vi "Finish.vi"   [LabVIEW 2016]
doc: "This VI is called just before exiting. It is expected to close I/O refnum, save collected data, etc."
uses:
  <vilib>/Rock Robotics/WPI/Utilities/WPI_GetSetVariantRefNum.vi
  <vilib>/Rock Robotics/WPI/Ultrasonic/WPI_SonarMB1010AnalogRefNum Registry Get.vi
  <vilib>/Rock Robotics/WPI/Ultrasonic/WPI_SonarMB1010AnalogClose.vi
types:
  T1 = typedef "WPI_SonarMB1010AnalogDeviceRef.ctl" = cluster{"AIDeviceRef":T2, "Scaling factor (V/in)":dbl, "Average Bits":u8}
  T2 = typedef "WPI_AnalogChannelDevRef.ctl" = cluster{"DevStatus":errorcluster, "Analog Channel":T3}
  T3 = typedef "FPGA_AIChannel.ctl" = enum8{"AI 0", "AI 1", "AI 2", "AI 3", "AI MXP 0", "AI MXP 1", "AI MXP 2", "AI MXP 3", "Invalid"}
  T4 = typedef "WPI_JoystickDevRef.ctl" = cluster{"Device":T5}
  T5 = typedef "WPI_JoystickDeviceEnum.ctl" = enum16{"USB 0", "USB 1", "USB 2", "USB 3", "USB 4", "USB 5"}
  T6 = typedef "WPI_RobotDriveDevRef.ctl" = cluster{"DevStatus":errorcluster, "Motors[]":T7[], "Square Inputs":bool, "Max Output":dbl}
  T7 = typedef "WPI_MotorControlDeviceRef.ctl" = cluster{"DeviceStatus":errorcluster, "Type":T8, "PWM":cluster{"PWM Channel":T9, "DeadBand":T10}, "CAN":cluster{"Device Number":u8, "SetOutput VI Ref":variant, "GetOutput VI Ref":variant, "Enable VI Ref":variant, "Disable VI Ref":variant, "Data":variant}, "Invert":bool}
  T8 = typedef "WPI_MotorControlType.ctl" = enum16{"PWM", "CAN"}
  T9 = typedef "FPGA_DIOPWMChannel.ctl" = enum8{"PWM 0", "PWM 1", "PWM 2", "PWM 3", "PWM 4", "PWM 5", "PWM 6", "PWM 7", "PWM 8", "PWM 9", "PWM MXP 0", "PWM MXP 1", "PWM MXP 2", "PWM MXP 3", "PWM MXP 4", "PWM MXP 5", "PWM MXP 6", "PWM MXP 7", "PWM MXP 8", "PWM MXP 9", "Invalid"}
  T10 = typedef "WPI_PWMDeadband.ctl" = cluster{"Name":string, "maxPositivePwm":i32, "minPositivePwm":i32, "centerPwm":i32, "maxNegativePwm":i32, "minNegativePwm":i32, "angularRange":u16}
  T11 = typedef "WPI_SwitchDevRef.ctl" = cluster{"DevStatus":errorcluster, "DIO Channel":T12, "CntIndex":T13, "Normally Closed":bool}
  T12 = typedef "FPGA_DIOChannel.ctl" = enum8{"DIO 0", "DIO 1", "DIO 2", "DIO 3", "DIO 4", "DIO 5", "DIO 6", "DIO 7", "DIO 8", "DIO 9", "DIO MXP 0", "DIO MXP 1", "DIO MXP 2", "DIO MXP 3", "DIO MXP 4", "DIO MXP 5", "DIO MXP 6", "DIO MXP 7", "DIO MXP 8", "DIO MXP 9", "DIO MXP 10", "DIO MXP 11", "DIO MXP 12", "DIO MXP 13", "DIO MXP 14", "DIO MXP 15", "SPI Port CS1", "SPI Port CS2", "SPI Port CS3", "SPI Port MISO", "SPI Port MOSI", "Invalid"}
  T13 = typedef "FPGA_CounterCtrSystemIndex.ctl" = enum8{"Ctr 0", "Ctr 1", "Ctr 2", "Ctr 3", "Ctr 4", "Ctr 5", "Ctr 6", "Ctr 7", "Invalid"}
  T14 = typedef "WPI_DigitalInputDevRef.ctl" = cluster{"DevStatus":errorcluster, "DIO Channel":T12}
  T15 = typedef "WPI_ServoDeviceRef.ctl" = cluster{"DeviceStatus":errorcluster, "PWM Channel":T9, "DeadBand":T10}
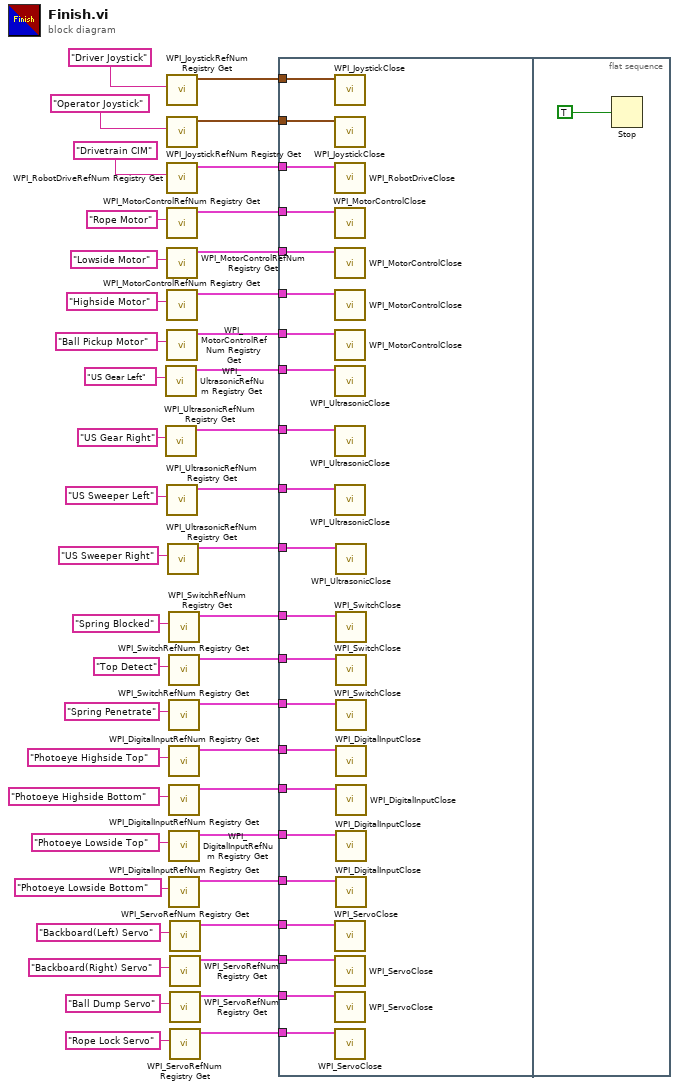
[diagram p0: block diagram]
diagram:
  n1 = call-poly <vilib>:"WPI_UltrasonicRefNum Registry Get.vi"("refnum name"="US Gear Left") -> ("SonarMB1010AnalogDevRef"=w30:T1)  [unwired: 9 in, 1 out]
  n2 = call-poly <vilib>:"WPI_UltrasonicRefNum Registry Get.vi"("refnum name"="US Gear Right") -> ("SonarMB1010AnalogDevRef"=w29:T1)  [unwired: 9 in, 1 out]
  n3 = call <vilib>:"WPI_JoystickRefNum Registry Get.vi"("refnum name"="Driver Joystick") -> ("JoystickDevRef"=w41:T4)  [unwired: 1 in, 9 out]
  n4 = call <vilib>:"WPI_JoystickRefNum Registry Get.vi"("refnum name"="Operator Joystick") -> ("JoystickDevRef"=w39:T4)  [unwired: 1 in, 9 out]
  n5 = call <vilib>:"WPI_RobotDriveRefNum Registry Get.vi"("refnum name"="Drivetrain CIM") -> ("RobotDriveDevRef"=w42:T6)  [unwired: 1 in, 9 out]
  n6 = call <vilib>:"WPI_MotorControlRefNum Registry Get.vi"("refnum name"="Rope Motor") -> ("MotorControlDevRef"=w34:T7)  [unwired: 9 in, 1 out]
  n7 = call <vilib>:"WPI_MotorControlRefNum Registry Get.vi"("refnum name"="Lowside Motor") -> ("MotorControlDevRef"=w33:T7)  [unwired: 9 in, 1 out]
  n8 = call <vilib>:"WPI_MotorControlRefNum Registry Get.vi"("refnum name"="Highside Motor") -> ("MotorControlDevRef"=w32:T7)  [unwired: 9 in, 1 out]
  n9 = call <vilib>:"WPI_MotorControlRefNum Registry Get.vi"("refnum name"="Ball Pickup Motor") -> ("MotorControlDevRef"=w31:T7)  [unwired: 9 in, 1 out]
  n10 = call-poly <vilib>:"WPI_UltrasonicRefNum Registry Get.vi"("refnum name"="US Sweeper Left") -> ("SonarMB1010AnalogDevRef"=w28:T1)  [unwired: 9 in, 1 out]
  n11 = call-poly <vilib>:"WPI_UltrasonicRefNum Registry Get.vi"("refnum name"="US Sweeper Right") -> ("SonarMB1010AnalogDevRef"=w27:T1)  [unwired: 9 in, 1 out]
  n12 = call <vilib>:"WPI_SwitchRefNum Registry Get.vi"("refnum name"="Spring Blocked") -> ("SwitchDevRef"=w22:T11)  [unwired: 9 in, 1 out]
  n13 = call <vilib>:"WPI_SwitchRefNum Registry Get.vi"("refnum name"="Top Detect") -> ("SwitchDevRef"=w21:T11)  [unwired: 9 in, 1 out]
  n14 = call <vilib>:"WPI_SwitchRefNum Registry Get.vi"("refnum name"="Spring Penetrate") -> ("SwitchDevRef"=w20:T11)  [unwired: 9 in, 1 out]
  n15 = call <vilib>:"WPI_DigitalInputRefNum Registry Get.vi"("refnum name"="Photoeye Highside Top") -> ("DigitalInputDevRef"=w16:T14)  [unwired: 9 in, 1 out]
  n16 = call <vilib>:"WPI_DigitalInputRefNum Registry Get.vi"("refnum name"="Photoeye Highside Bottom") -> ("DigitalInputDevRef"=w15:T14)  [unwired: 9 in, 1 out]
  n17 = call <vilib>:"WPI_DigitalInputRefNum Registry Get.vi"("refnum name"="Photoeye Lowside Top") -> ("DigitalInputDevRef"=w14:T14)  [unwired: 9 in, 1 out]
  n18 = call <vilib>:"WPI_DigitalInputRefNum Registry Get.vi"("refnum name"="Photoeye Lowside Bottom") -> ("DigitalInputDevRef"=w9:T14)  [unwired: 9 in, 1 out]
  n19 = call <vilib>:"WPI_ServoRefNum Registry Get.vi"("refnum name"="Backboard(Left) Servo") -> ("ServoDeviceRef"=w8:T15)  [unwired: 9 in, 1 out]
  n20 = call <vilib>:"WPI_ServoRefNum Registry Get.vi"("refnum name"="Backboard(Right) Servo") -> ("ServoDeviceRef"=w7:T15)  [unwired: 9 in, 1 out]
  n21 = call <vilib>:"WPI_ServoRefNum Registry Get.vi"("refnum name"="Ball Dump Servo") -> ("ServoDeviceRef"=w6:T15)  [unwired: 9 in, 1 out]
  n22 = call <vilib>:"WPI_ServoRefNum Registry Get.vi"("refnum name"="Rope Lock Servo") -> ("ServoDeviceRef"=w5:T15)  [unwired: 9 in, 1 out]
  n23 = flat-sequence {
    tunnel: w42 -> [w66]
    tunnel: w41 -> [w65]
    tunnel: w39 -> [w64]
    tunnel: w34 -> [w63]
    tunnel: w33 -> [w62]
    tunnel: w32 -> [w61]
    tunnel: w31 -> [w60]
    tunnel: w30 -> [w59]
    tunnel: w29 -> [w58]
    tunnel: w28 -> [w57]
    tunnel: w27 -> [w56]
    tunnel: w22 -> [w55]
    tunnel: w21 -> [w54]
    tunnel: w20 -> [w53]
    tunnel: w16 -> [w52]
    tunnel: w15 -> [w51]
    tunnel: w14 -> [w50]
    tunnel: w9 -> [w49]
    tunnel: w8 -> [w48]
    tunnel: w7 -> [w47]
    tunnel: w6 -> [w46]
    tunnel: w5 -> [w45]
    frame #0 {
      n24 = call <vilib>:"WPI_JoystickClose.vi"("JoystickDevRef"=w65) -> ()  [unwired: 11 out]
      n25 = call <vilib>:"WPI_JoystickClose.vi"("JoystickDevRef"=w64) -> ()  [unwired: 11 out]
      n26 = call <vilib>:"WPI_RobotDriveClose.vi"("RobotDriveDevRef"=w66) -> ()  [unwired: 1 in, 10 out]
      n27 = call <vilib>:"WPI_MotorControlClose.vi"("MotorControlDevRef"=w63) -> ()  [unwired: 10 in, 1 out]
      n28 = call <vilib>:"WPI_MotorControlClose.vi"("MotorControlDevRef"=w62) -> ()  [unwired: 10 in, 1 out]
      n29 = call <vilib>:"WPI_MotorControlClose.vi"("MotorControlDevRef"=w61) -> ()  [unwired: 10 in, 1 out]
      n30 = call <vilib>:"WPI_MotorControlClose.vi"("MotorControlDevRef"=w60) -> ()  [unwired: 10 in, 1 out]
      n31 = call-poly <vilib>:"WPI_UltrasonicClose.vi"("SonarMB1010AnalogDevRef"=w59) -> ()  [unwired: 10 in, 1 out]
      n32 = call-poly <vilib>:"WPI_UltrasonicClose.vi"("SonarMB1010AnalogDevRef"=w58) -> ()  [unwired: 10 in, 1 out]
      n33 = call-poly <vilib>:"WPI_UltrasonicClose.vi"("SonarMB1010AnalogDevRef"=w57) -> ()  [unwired: 10 in, 1 out]
      n34 = call <vilib>:"WPI_ServoClose.vi"("ServoDeviceRef"=w48) -> ()  [unwired: 10 in, 1 out]
      n35 = call <vilib>:"WPI_ServoClose.vi"("ServoDeviceRef"=w47) -> ()  [unwired: 10 in, 1 out]
      n36 = call <vilib>:"WPI_ServoClose.vi"("ServoDeviceRef"=w46) -> ()  [unwired: 10 in, 1 out]
      n37 = call <vilib>:"WPI_ServoClose.vi"("ServoDeviceRef"=w45) -> ()  [unwired: 10 in, 1 out]
      n38 = call-poly <vilib>:"WPI_UltrasonicClose.vi"("SonarMB1010AnalogDevRef"=w56) -> ()  [unwired: 10 in, 1 out]
      n39 = call <vilib>:"WPI_SwitchClose.vi"("SwitchDevRef"=w55) -> ()  [unwired: 10 in, 1 out]
      n40 = call <vilib>:"WPI_SwitchClose.vi"("SwitchDevRef"=w54) -> ()  [unwired: 10 in, 1 out]
      n41 = call <vilib>:"WPI_SwitchClose.vi"("SwitchDevRef"=w53) -> ()  [unwired: 10 in, 1 out]
      n42 = call <vilib>:"WPI_DigitalInputClose.vi"("DigitalInputDevRef"=w52) -> ()  [unwired: 10 in, 1 out]
      n43 = call <vilib>:"WPI_DigitalInputClose.vi"("DigitalInputDevRef"=w51) -> ()  [unwired: 10 in, 1 out]
      n44 = call <vilib>:"WPI_DigitalInputClose.vi"("DigitalInputDevRef"=w50) -> ()  [unwired: 10 in, 1 out]
      n45 = call <vilib>:"WPI_DigitalInputClose.vi"("DigitalInputDevRef"=w49) -> ()  [unwired: 10 in, 1 out]
    }
    frame #1 {
      n46 = Stop(stop? (T)=TRUE ("Quit")) -> ()
    }
  }
